vi "TA_Open_TA.vi"(11 "Path":path=path "/Users/tm/Desktop/fs-TA/Data/demo_fsta.dat") -> (2 "Size (Raw TA)":i32[](array[numeric]), 3 "Raw TA":dbl[][](array[numeric]) format="%#_8g")   [LabVIEW 2025]
uses:
  <vilib>/Utility/file.llb/Read Delimited Spreadsheet (DBL).vi
panel:
  in  "App:Default Data Directory":path
  in  "Application Directory":path
  in  "delimiter (\\t tab; , comma)":string="\t"
  in  "transpose? (F)":bool
  in  "max characters/row  (no limit:0)":i32
  in  "start of read offset (chars.:0)":i32
  in  "number of rows (all:-1)":i32=-1
  in  "format (%.10f)":string="%.10f"
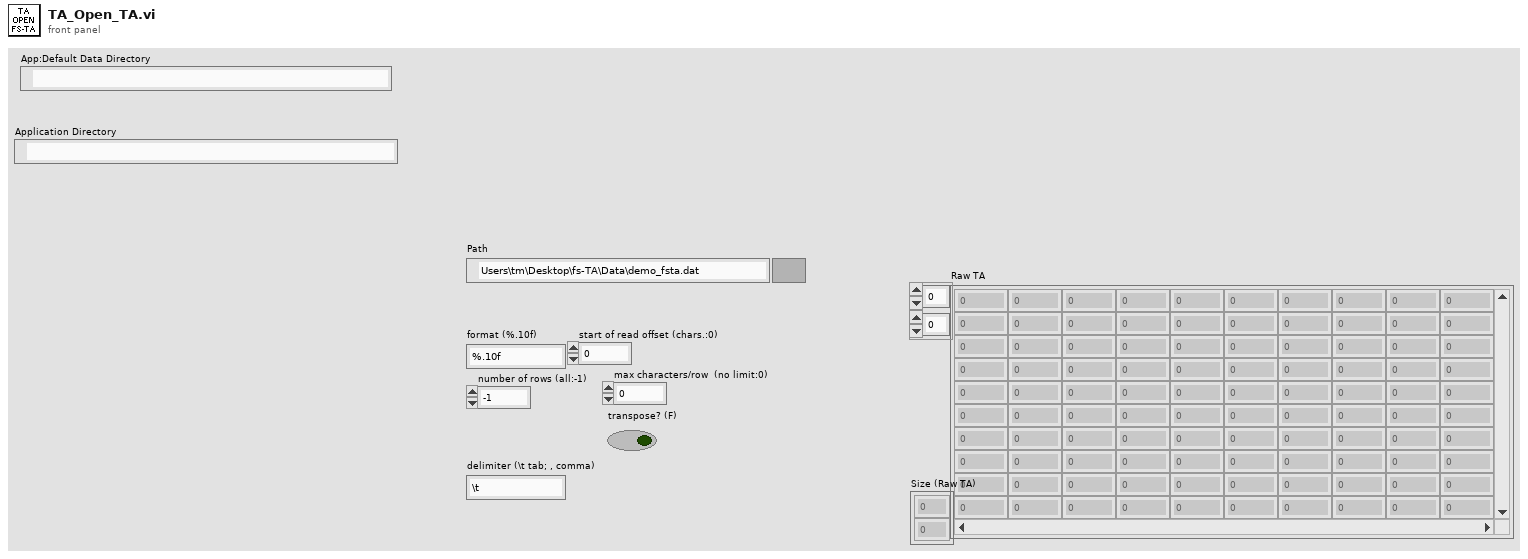
[diagram p1: front panel]
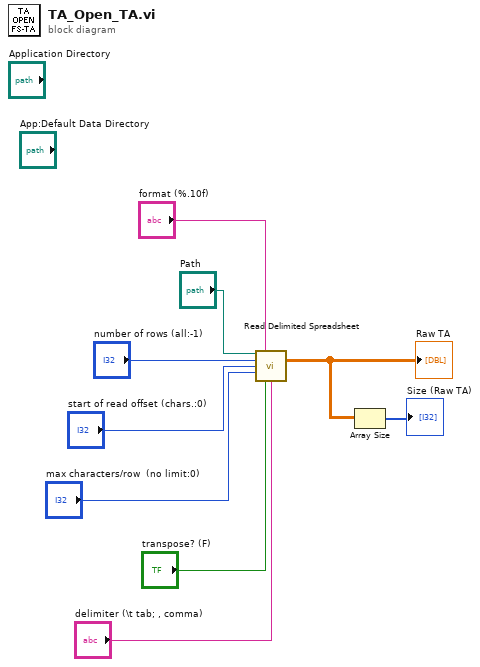
[diagram p0: block diagram]
diagram:
  n1 = call-poly <vilib>:"Read Delimited Spreadsheet.vi"("file path (dialog if empty)"="Path", "format (%.3f)"="format (%.10f)", "number of rows (all:-1)"="number of rows (all:-1)", "start of read offset (chars.:0)"="start of read offset (chars.:0)", "max characters/row  (no limit:0)"="max characters/row  (no limit:0)", "transpose? (F)"="transpose? (F)", "delimiter (\\t)"="delimiter (\\t tab; , comma)") -> ("all rows"=w2:dbl[][])  [unwired: 3 in, 5 out]
  "Raw TA" <- w2
  n2 = Array Size(array=w2) -> (size(s)=→"Size (Raw TA)":i32[])
